vi "Actor Core.vi"(8 "error in":errorcluster, 11 "Fault Monitor in":refnum<class "Fault Monitor.lvclass">) -> (0 "error out":errorcluster, 3 "Actor out":refnum<class "Actor.lvclass">)   [LabVIEW 2023, in "Fault Monitor.lvlib" / "Fault Monitor.lvclass"]
doc: "Base Class for the bottom subpanel.\nThis provides the basic implementation for show/hide operations.\n\nancestor classes should override this, but maintain proportions."
uses:
  Library/Fault Monitor.lvclass
  builds/Framework/Actor Framework.lvlibp/1abvi3w/vi.lib/ActorFramework/Actor/Actor.lvclass
  Fault Monitor Messages/Handle Faults Msg/Handle Faults Msg.lvclass/Handle Faults Msg.ctl
  Fault Monitor Messages/Clear Target Faults Msg/Clear Target Faults Msg.lvclass/Clear Target Faults Msg.ctl
  builds/Framework/Actor Framework.lvlibp/1abvi3w/vi.lib/ActorFramework/Message Enqueuer/Enqueue.vi
  Fault Monitor Messages/Handle Faults Msg/Handle Faults Msg.lvclass
  Fault Monitor Messages/Clear Target Faults Msg/Clear Target Faults Msg.lvclass
  builds/Main/Docking.lvlibp/Bottom Panel/BottomDock.lvclass
  builds/Framework/Engine.lvlibp/Engine/Library/Engine.lvclass
  C:/Users/Public/Documents/Development/builds/Framework/Engine.lvlibp/Engine/Library/Engine.lvclass
panel:
  in  "Warnings":bool
  out "Warning History":string
  in  "Active Warnings":i32(listbox)
  in  "Errors":bool
  out "Error History":string
  in  "Active Errors":i32(listbox)
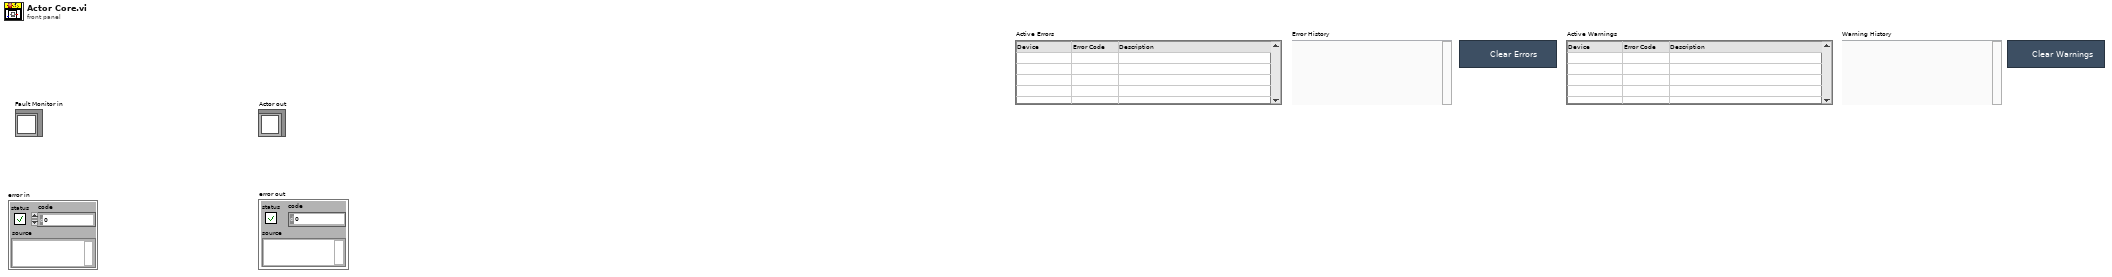
[diagram p1: front panel]
types:
  T1 = cluster{"Pnl Actor":refnum<event-registration>, "Event Registration Refnum":refnum<event-registration>}
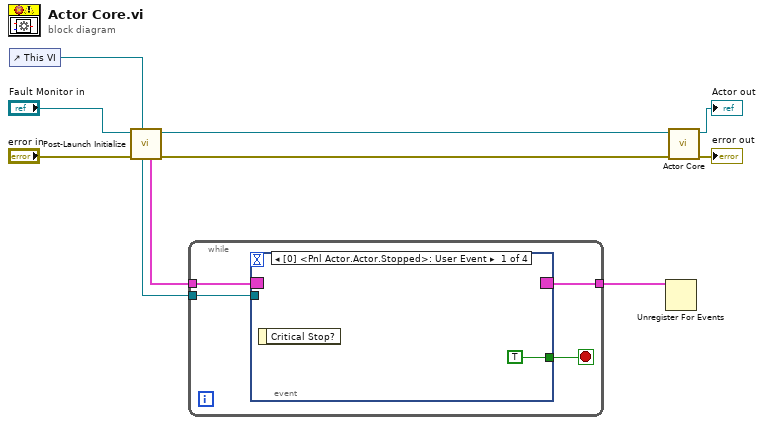
[diagram p0: block diagram]
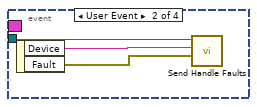
[diagram p2: hidden frame]
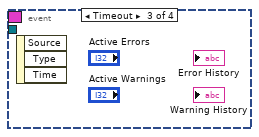
[diagram p3: hidden frame]
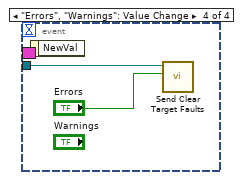
[diagram p4: hidden frame]
diagram:
  n1 = control-ref of="This VI"() -> (w2:refnum<vi>)
  n2 = call "Post-Launch Initialize.vi"("GUI Reference"=w2, "error in (no error)"="error in", "Engine in"="Fault Monitor in") -> ("error out"=w4:errorcluster, "Engine out"=w6:refnum<class "Fault Monitor.lvclass">, "Registered Events"=w1:T1, "Self Enqueuer"=w3:refnum<class "Message Enqueuer.lvclass">)  [unwired: 5 in]
  n3 = while {
    tunnel: w3 -> [w13]
    tunnel: [w11] -> w8
    tunnel: w1 -> [w12]
    stop <- w14 stop-if-true
    n4 = event shown="[0] <Pnl Actor.Actor.Stopped>: User Event" {
      selector: w12 -> [_ _ _ _]
      dyn-events: [_ _ _ _] -> w11
      timeout: _ -> [_ _ _ _]
      tunnel: [TRUE _ _ _] -> w14
      tunnel: w13 -> [_ w18 _ w20]
      event User Event {
        n5 = event-data() -> ()  [unwired: 1 in, 1 out]
      }
      event User Event {
        n6 = event-data() -> ("Device"=w17:string, "Fault"=w16:errorcluster)  [unwired: 1 in]
        n7 = call "Send Handle Faults.vi"("Fault"=w16, "Device"=w17, "Message Enqueuer"=w18) -> ()  [unwired: 7 in, 2 out]
      }
      event Timeout {
        n8 = event-data() -> ()  [unwired: 1 in, 3 out]
      }
      event "Errors", "Warnings": Value Change {
        n9 = event-data() -> ()  [unwired: 1 in, 1 out]
        n10 = call "Send Clear Target Faults.vi"("Clear Alarms"="Errors", "Message Enqueuer"=w20) -> ()  [unwired: 8 in, 2 out]
      }
    }
  }
  n11 = Unregister For Events(event registration refnum=w8) -> ()  [unwired: 1 in, 1 out]
  n12 = call-parent "Actor Core.vi"("error in"=w4, "Bottom Panel in"=w6) -> ("error out"=→"error out":errorcluster, "Actor out"=→"Actor out":refnum<class "Actor.lvclass">)  [unwired: 8 in]
